vi "select actions list vi dialog.vi"(8 "error in (no error)":errorcluster, 11 "sequencer configuration":refnum<class "Simple Sequencer TBM configuration.lvclass">) -> (0 "error out":errorcluster, 1 "success?":bool, 2 "supported actions list":T1[](array[typedef]), 3 "sequencer configuration out":refnum<class "Simple Sequencer TBM configuration.lvclass">)   [LabVIEW 2014, in "Simple Sequencer TBM editor node.lvclass"]
doc: "This is a dialog that allows users to specify the location of a VI that defines the actions supported by this instance of the sequencer."
uses:
  Simple Sequencer TBM editor node.lvclass
  module/configuration/Simple Sequencer TBM configuration.lvclass
  action config and UI pairing.ctl
  sequencer parent classes/action configuration parent/action configuration.lvclass
  module/configuration/Simple Sequencer TBM configuration.lvclass/Simple Sequencer TBM configuration.ctl
  module/configuration/Write supported actions list VI.vi
  module/configuration/Read supported actions list VI.vi
  supported actions list template.vi
panel:
  in  "Cancel Button":bool
  in  "OK Button":bool
  in  "File Path Control":path
  # "This VI's connector pane must match the 'supported actions list template.vi' located in the 'Simple Sequencer TBM editor node.lvclass'."
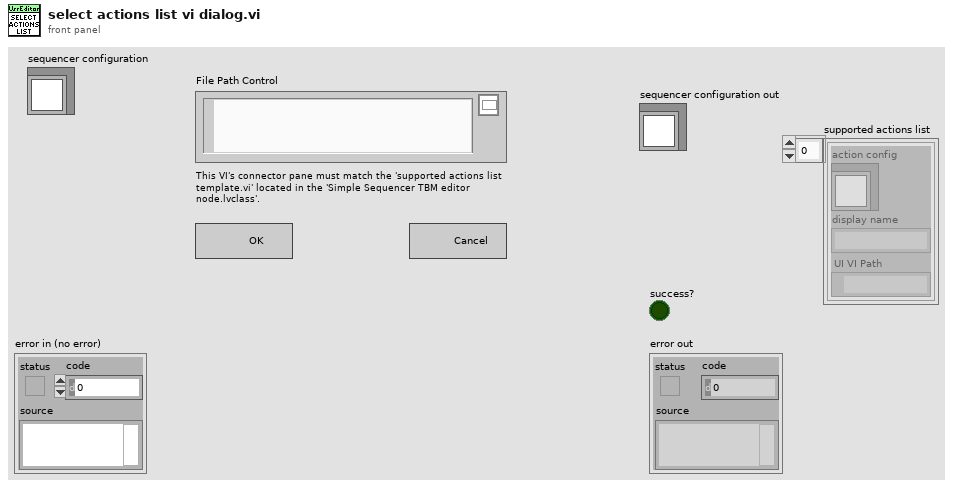
[diagram p1: front panel]
types:
  T1 = typedef "Simple Sequencer TBM editor node.lvclass/action config and UI pairing.ctl" = cluster{"action config":refnum<class "action configuration.lvclass">, "display name":string, "UI VI Path":path}
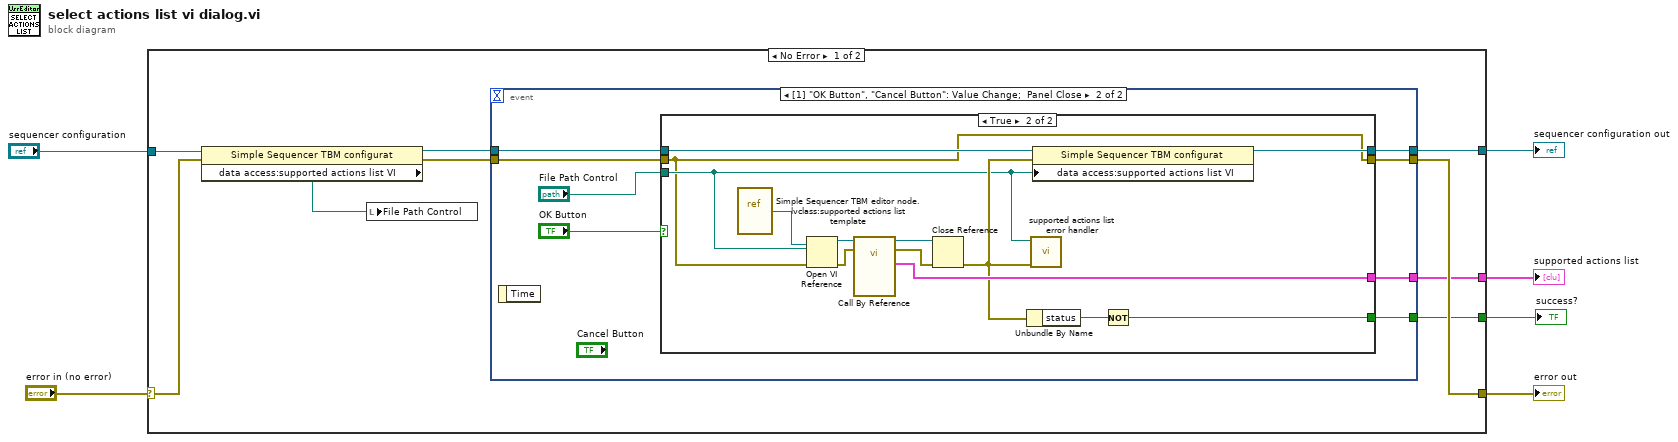
[diagram p0: block diagram]
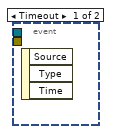
[diagram p2: hidden frame]
diagram:
  n1 = case shown="No Error" "error in (no error)" {
    selector: "error in (no error)" -> [w14 w40]
    tunnel: [w9 w40] -> w5
    tunnel: "sequencer configuration" -> [w15 w39]
    tunnel: [w10 w39] -> w3
    tunnel: [w8 _] -> w1
    tunnel: [w7 _] -> w2
    frame No Error {
      n2 = property class="Simple Sequencer TBM configurat"(reference=w15, error in=w14) -> (reference out=w12:refnum<class "Simple Sequencer TBM configuration.lvclass">, error out=w11:errorcluster, "data access:supported actions list VI"=w13:path)
      n3 = local write "File Path Control"(w13) -> ()
      n4 = event shown="[1] \"OK Button\", \"Cancel Button\": Value Change;  Panel Close" {
        selector: _ -> [_ _]
        dyn-events: _ -> [_ _]
        timeout: _ -> [_ _]
        tunnel: w12 -> [_ w22]
        tunnel: w11 -> [_ w21]
        tunnel: [_ w19] -> w9
        tunnel: [_ w18] -> w10
        tunnel: [_ w17] -> w8
        tunnel: [_ w16] -> w7
        event Timeout {
          n5 = event-data() -> ()  [unwired: 1 in, 3 out]
        }
        event "OK Button", "Cancel Button": Value Change; Panel Close {
          n6 = event-data() -> ()  [unwired: 1 in, 1 out]
          n7 = case shown="True" "OK Button" {
            tunnel: w22 -> [w25 w38]
            tunnel: w21 -> [w24 w26]
            tunnel: "File Path Control" -> [_ w27]
            tunnel: [w24 w26] -> w19
            tunnel: [w25 w37] -> w18
            tunnel: [_ w32] -> w17
            tunnel: [_ w30] -> w16
            frame False {
            }
            frame True {
              n8 = vi-ref "Simple Sequencer TBM editor node.lvclass:supported actions list template.vi"() -> (w29:refnum<vi>)
              n9 = Open VI Reference(type specifier VI Refnum (for type only)=w29, vi path=w27, error in (no error)=w26) -> (vi reference=w35:refnum<vi>, error out=w34:errorcluster)  [unwired: 3 in]
              n10 = call-by-ref "?"(reference=w35, error in=w34) -> (reference out=w36:refnum<vi>, error out=w33:errorcluster, "supported actions list"=w32:T1[])  [unwired: 11 in]
              n11 = Close Reference(reference=w36, error in (no error)=w33) -> (error out=w28:errorcluster)
              n12 = Unbundle By Name(w28) -> ("status"=w31:bool)
              n13 = call "supported actions list error handler.vi"("error in (no error)"=w28, "Path"=w27) -> ()  [unwired: 10 in]
              n14 = property class="Simple Sequencer TBM configurat"(reference=w38, error in=w28, "data access:supported actions list VI"=w27) -> (reference out=w37:refnum<class "Simple Sequencer TBM configuration.lvclass">)  [unwired: 1 out]
              n15 = Not(x=w31) -> (.not. x?=w30:bool)
            }
          }
        }
      }
    }
    frame Error {
    }
  }
  "error out" <- w5
  "sequencer configuration out" <- w3
  "supported actions list" <- w1
  "success?" <- w2
